vi "SVFA Zoom Power Spectrum (N Ch).vi"(0 "scaled signals [EU]":waveform(dbl)[](array[waveform]), 3 "zoom settings":T2={"frequency range"={"start frequency"=1000.0, "stop frequency"=2000.0}, "window"=1, "number of lines"=400, "% overlap"=0.0} {"% overlap" min=0.0 format="%.2f"; "number of lines" min=2; "window" items=["None ", "Hanning", "Hamming", "Blackman-Harris", "Exact Blackman", "Blackman", "Flat Top", "4 Term B-Harris ", "7 Term B-Harris", "Low Sidelobe"]; "frequency range"."stop frequency" min=0.0 format="%.2f"; "frequency range"."start frequency" min=0.0 format="%.2f"}, 4 "dB On (T)":bool=TRUE, 5 "error in (no error)":errorcluster, 7 "averaging parameters":T1={"averaging mode"=enum."No averaging", "weighting mode"=enum."Exponential", "number of averages"=10, "linear mode"=enum."One shot"} {"number of averages" min=1 step=1}, 9 "restart averaging (F)":bool) -> (11 "averaging done":bool, 12 "new spectrum available":bool, 13 "averages completed":dbl, 14 "power spectra [dB EU]":cluster{"f0":dbl, "df":dbl, "magnitude":dbl[]}[](array[cluster]) {"magnitude" format="%.2p"; "df" format="%.2p"; "f0" format="%.2p"}, 15 "unit labels":string[](array[string]), 18 "spectrum info":T3[](array[typedef]) {"x-axis units" items=["Time (s)"=0, "Frequency-CB (Hz)"=1, "Frequency-CPB (Hz)"=1248, "Frequency-Arbitrary (Hz)"=2357, "Quefrency (s)"=2, "Revolutions (rev)"=3, "Order"=4, "Speed (RPM)"=11, "Speed (rad/s)"=21, "Index"=65535]; "weighting filter" items=["Linear", "A-weighting", "B-weighting", "C-weighting", "ITU-R 468-4", "Dolby", "CCITT", "C-message", "Wb", "Wc", "Wd", "We", "Wf", "Wh", "Wj", "Wk", "Wm", "AES17 20 kHz lowpass", "AES17 40 kHz lowpass", "AES17 20 kHz highpass", "AES17 40 kHz highpass"]; "dB reference [EU]" format="%.2f"; "engineering units" items=["custom..."=0, "V"=1, "A"=21, "C"=30, "pC"=31, "s"=32, "-"=29, "Pa"=2, "N"=20, "g"=3, "m/s^2"=4, "m/s"=5, "m"=6, "mm/s"=12, "mm"=13, "micron/s"=14, "micron"=15, "in/s^2"=7, "in/s"=8, "in"=9, "mil/s"=10, "mil"=11, "rad/s^2"=16, "rad/s"=17, "rad"=18, "deg/s^2"=26, "deg/s"=27, "deg"=28, "RPM"=22, "cycle/s^2"=23, "Hz"=24, "cycle"=25, "strain"=19]; "spectral info"."window" items=["None "=0, "Hanning"=1, "Hamming"=2, "Blackman-Harris"=3, "Exact Blackman"=4, "Blackman"=5, "Flat Top"=6, "4 Term B-Harris "=7, "7 Term B-Harris"=8, "Low Sidelobe"=9, "Force - Exponential"=10, "Gaussian"=62]}, 19 "error out":errorcluster)   [LabVIEW 2017]
doc: "Computes the zoom power spectrum of <B>scaled signal [EU]</B> and <B>zoom settings</B>. Data accumulates each time this VI is called. However, it returns a new spectrum only when sufficient data accumulates. Indicators and subsequent processing should only be called when <B>new spectrum available</B> is TRUE. Wire data to the <B>scaled signal [EU]</B> input to determine the polymorphic instance to use or manually select the instance."
uses:
  <vilib>/addons/_NISVFA/_Shared subVIs/Controls/svc_Spectrum Info.ctl
  <vilib>/addons/_NISVFA/_Shared subVIs/Controls/svc_X-Axis Units.ctl
  <vilib>/addons/_NISVFA/_Shared subVIs/Controls/svc_Spectrum Type.ctl
  <vilib>/addons/_NISVFA/_Shared subVIs/Controls/svc_Engineering Units Text Ring.ctl
  <vilib>/addons/_NISVFA/_Shared subVIs/Controls/svc_Weighting Filter Text Ring.ctl
  <vilib>/addons/_NISVFA/_Shared subVIs/Controls/svc_Complimentary Spectrum Units.ctl
  <vilib>/addons/_NISVFA/_Shared subVIs/Spectrum Info/svfa_Build Spectrum Info.vi
  <vilib>/addons/_NISVFA/_Shared subVIs/Spectrum Averaging/svfa_Reset Averaging State Info.vi
  <vilib>/addons/_NISVFA/_Shared subVIs/Spectrum Averaging/svfa_Average Array with Avg Checks (complex) No State.vi
  <vilib>/addons/_NISVFA/_Shared subVIs/Common/svc_Complex to Mag2 Array.vi
  <vilib>/addons/_NISVFA/_Shared subVIs/Spectrum Averaging/svfa_Average Array with Avg Checks (real) No State.vi
  <vilib>/addons/_NISVFA/_Shared subVIs/Common/svc_Get SV Channel Info.vi
  <vilib>/addons/_NISVFA/_Shared subVIs/Common/svc_Spectrum Units.vi
  <vilib>/addons/_NISVFA/_Shared subVIs/Spectrum Averaging/svfa_Average Array (complex) No State.vi
  <vilib>/addons/_NISVFA/_Shared subVIs/Spectrum Averaging/svfa_Average Array (real) No State.vi
  <vilib>/addons/_NISVFA/_Shared subVIs/Spectrum Averaging/svfa_No Average Array (complex).vi
  <vilib>/addons/_NISVFA/_Shared subVIs/Spectrum Averaging/svfa_Average Array (complex).vi
  <vilib>/addons/_NISVFA/_Shared subVIs/Spectrum Averaging/svfa_No Average Array (real).vi
  <vilib>/addons/_NISVFA/_Shared subVIs/Spectrum Averaging/svfa_Average Array (real).vi
  <vilib>/addons/_NISVFA/_Shared subVIs/Spectrum Averaging/svfa_Peak Hold Array.vi
  <vilib>/addons/_NISVFA/_Shared subVIs/Common/svc_Get Weighting Enum and Labels.vi
  <vilib>/addons/_NISVFA/_Shared subVIs/Common/svc_Unit Label Lexical Class.vi
  <vilib>/addons/_NISVFA/_Shared subVIs/Common/svc_Engineering Units to Unit Label.vi
  <vilib>/addons/_NISVFA/_Shared subVIs/Common/svc_Format Value (DBL).vi
  <vilib>/addons/_NISVFA/_Shared subVIs/Common/svc_Channel Info to Spectrum Info.vi
  <vilib>/addons/_NISVFA/_Shared subVIs/Common/svc_Unit Label to Engineering Units.vi
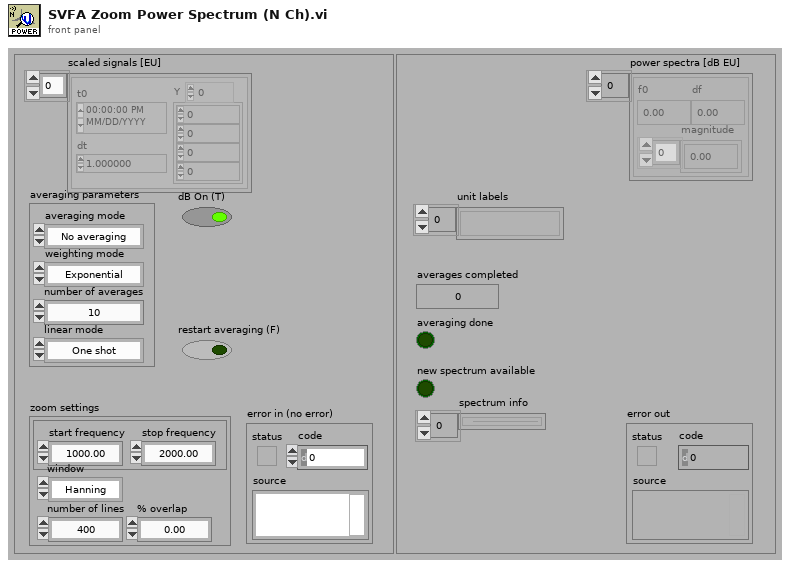
[diagram p1: front panel]
types:
  T1 = cluster{"averaging mode":enum16{"No averaging", "Vector averaging", "RMS averaging", "Peak hold"}, "weighting mode":enum16{"Linear", "Exponential"}, "number of averages":u32, "linear mode":enum16{"One shot", "Auto restart"}}
  T2 = cluster{"frequency range":cluster{"start frequency":dbl, "stop frequency":dbl}, "window":u16, "number of lines":i32, "% overlap":dbl}
  T3 = typedef "svc_Spectrum Info.ctl" = cluster{"channel name":string, "description":string, "x-axis units":T4, "spectral info":cluster{"spectrum type":T5, "linear/dB":enum16{"linear", "dB"}, "window":u16, "window size":i32, "FFT size":i32}, "engineering units":T6, "custom label":string, "dB reference [EU]":dbl, "peak units":enum16{"rms", "peak", "peak-peak"}, "weighting filter":T7, "spectral density?":bool, "unit label":string, "spectrum skewed?":bool, "complimentary spectrum units":T8}
  T4 = typedef "svc_X-Axis Units.ctl" = u16
  T5 = typedef "svc_Spectrum Type.ctl" = enum16{"FFT Spectrum [complex]", "Amplitude [Magnitude]", "Power [Magnitude^2]", "Cross Spectrum [complex]", "Frequency Response [Complex]"}
  T6 = typedef "svc_Engineering Units Text Ring.ctl" = u16
  T7 = typedef "svc_Weighting Filter Text Ring.ctl" = u16
  T8 = typedef "svc_Complimentary Spectrum Units.ctl" = enum16{"none", "radians", "degrees", "cycles", "imaginary"}
  T9 = enum16{"Restart processing", "Continue processing", "Skip processing"}
  T10 = enum16{"No averaging", "Vector averaging", "RMS averaging", "Peak hold"}
  T11 = cluster{"complex FFT":cdb[], "real FFT":dbl[], "f0":dbl, "df":dbl, "averages completed":dbl, "averaging parameters":cluster{"averaging mode":enum16{"No averaging", "Vector averaging", "RMS averaging", "Peak hold"}, "weighting mode":enum16{"Linear", "Exponential"}, "number of averages":u32, "linear mode":enum16{"One shot", "Auto restart"}}}[]
  T12 = cluster{"zoom settings":cluster{"center frequency":dbl, "zoom":i32, "trim":dbl}, "FFT settings":cluster{"window":enum16{"None ", "Hanning", "Hamming", "Blackman-Harris", "Exact Blackman", "Blackman", "Flat Top", "4 Term B-Harris ", "7 Term B-Harris", "Low Sidelobe"}, "window size":i32, "FFT size":i32, "%overlap":dbl}}
  T13 = cluster{"complex FFT":cdb[], "real FFT":dbl[], "f0":dbl, "df":dbl, "averages completed":dbl, "averaging parameters":cluster{"averaging mode":enum16{"No averaging", "Vector averaging", "RMS averaging", "Peak hold"}, "weighting mode":enum16{"Linear", "Exponential"}, "number of averages":u32, "linear mode":enum16{"One shot", "Auto restart"}}}
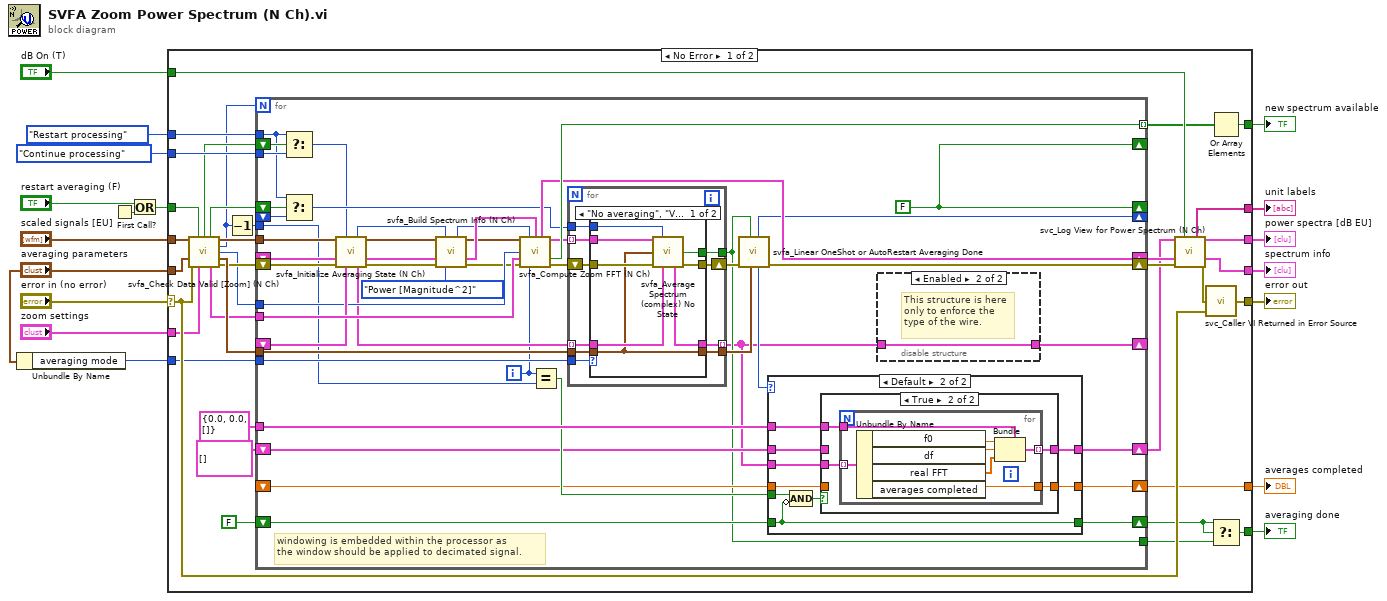
[diagram p0: block diagram]
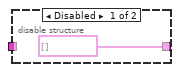
[diagram p2: hidden frame]
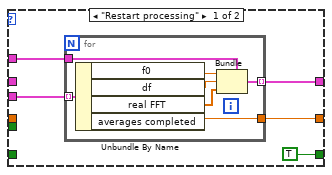
[diagram p3: hidden frame]
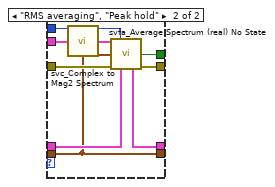
[diagram p5: hidden frame]
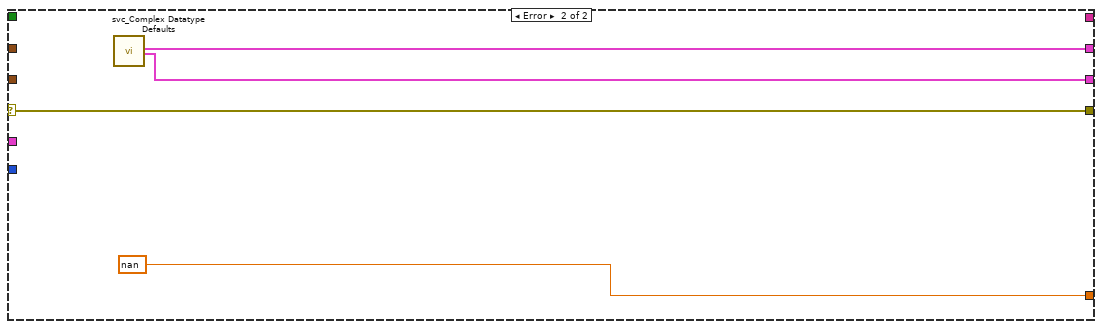
[diagram p6: hidden frame]
diagram:
  n1 = Unbundle By Name("averaging parameters") -> ("averaging mode"=w1:T10)
  n2 = First Call?() -> (First Call?: T/F=w7:bool)
  n3 = Or(x="restart averaging (F)", y=w7) -> (x .or. y?=w5:bool)
  n4 = case shown="No Error" "error in (no error)" {
    selector: "error in (no error)" -> [w37 w167]
    tunnel: w5 -> [w31 _]
    tunnel: [w23 nan ("Averaged So-far")] -> w18
    tunnel: [w34 _] -> w17
    tunnel: [w52 w164] -> w13
    tunnel: [w46 w167] -> w16
    tunnel: "averaging parameters" -> [w47 _]
    tunnel: "zoom settings" -> [w36 _]
    tunnel: "scaled signals [EU]" -> [w53 _]
    tunnel: [w50 _] -> w12
    tunnel: "dB On (T)" -> [w49 _]
    tunnel: [w48 w165] -> w11
    tunnel: [w22 _] -> w9
    tunnel: T9."Restart processing" ("processing control in") -> [w33 _]
    tunnel: T9."Continue processing" ("processing control in") -> [w32 _]
    tunnel: w1 -> [w29 _]
    frame No Error {
      n5 = call <vilib>:"svfa_Check Data Valid [Zoom] (N Ch).vi"("scaled signals [EU]"=w53, "restart averaging (F)"=w31, "averaging parameters"=w47, "error in (no error)"=w37, "zoom settings"=w36) -> ("reset processing"=w30:bool, "restart averaging"=w38:bool, "dup scaled signals"=w44:waveform(dbl)[], "iterations"=w28:i32, "maximum block size"=w35:i32, "dup averaging parameters"=w41:T1, "zoom FFT settings"=w39:T12, "error out"=w40:errorcluster)  [unwired: 3 in]
      n6 = Decrement(x=w28) -> (x-1=w27:i32)
      n7 = for {
        N: w28 -> [_]
        tunnel: [w97] -> w45 mode=indexing
        tunnel: w39 -> [w99]
        tunnel: w44 -> [w100]
        tunnel: [w56] -> w21
        shift-left: _ -> [w93]
        shift-right: [w54] -> _
        shift-right: [w95] -> w43
        shift-left: _ -> [w94]
        tunnel: w41 -> [w92]
        shift-right: [w60] -> _
        shift-left: _ -> [w91]
        shift-right: [w67] -> _
        shift-left: w38 -> [w89]
        tunnel: w35 -> [w88]
        shift-right: [w96] -> w42
        shift-left: w40 -> [w98]
        tunnel: w33 -> [w85]
        tunnel: w32 -> [w87]
        tunnel: w29 -> [w83]
        tunnel: w27 -> [w68]
        shift-right: [w67] -> _
        shift-left: w30 -> [w86]
        tunnel: cluster{"f0":dbl, "df":dbl, "real FFT":dbl[]} {"f0"=0.0, "df"=0.0, "real FFT"=[]} ("cluster") -> [w66]
        shift-right: [w64] -> w23
        shift-left: _ -> [w61]
        shift-right: [w63] -> w20
        shift-left: FALSE ("restart averaging") -> [w62]
        shift-right: [w58] -> w24
        shift-left: cluster{"f0":dbl, "df":dbl, "real FFT":dbl[]}[] [] -> [w57]
        i -> [w59]
        w67 = FALSE ("restart averaging")
        # "windowing is embedded within the processor as \nthe window should be applied to decimated signal."
        n8 = Select(t=w85, s=w86, f=w87) -> (s? t:f=w84:T9)
        n9 = Select(t=w85, s=w89, f=w91) -> (s? t:f=w90:T9)
        n10 = call <vilib>:"svfa_Initialize Averaging State (N Ch).vi"("Windowed Waveform(s)"=w100, "processing control in"=w84, "spectra info in"=w94, "error in (no error)"=w98, "state info"=w93) -> ("processing control out"=w77:T9, "Windowed Waveform(s)"=w76:waveform(dbl)[], "spectra info out"=w74:T3[], "state info"=w73:T11, "error out"=w75:errorcluster)  [unwired: 6 in]
        n11 = call <vilib>:"svfa_Build Spectrum Info (N Ch).vi"("scaled signal(s)"=w76, "processing control in"=w77, "spectra info in"=w74, "error in (no error)"=w75, "spectrum type"=svc_Spectrum_Type."Power [Magnitude^2]") -> ("dup processing control"=w70:T9, "dup scaled signals"=w79:waveform(dbl)[], "spectra info out"=w81:T3[], "error out"=w71:errorcluster)  [unwired: 7 in]
        n12 = call <vilib>:"svfa_Compute Zoom FFT (N Ch).vi"("scaled signals [EU]"=w79, "processing control"=w70, "spectra info in"=w81, "maximum block size"=w88, "zoom FFT settings"=w99, "error in (no error)"=w71, "iteration"=w59) -> ("spectra info out"=w95:T3[], "FFT spectra"=w78:cluster{"f0":dbl, "df":dbl, "spectrum":cdb[]}[], "spectrum ready"=w97:bool, "error out"=w80:errorcluster)  [unwired: 4 in, 1 out]
        n13 = Equal?(x=w59, y=w68) -> (x = y?=w65:bool)
        n14 = for {
          tunnel: [w146] -> w56
          tunnel: w78 -> [w145] mode=indexing
          tunnel: w90 -> [w142]
          tunnel: w92 -> [w141]
          tunnel: w83 -> [w140]
          tunnel: w73 -> [w139] mode=indexing
          tunnel: [w138] -> w55 mode=indexing
          shift-right: [w143] -> w82
          shift-left: w80 -> [w144]
          tunnel: [w137] -> w69
          n15 = case shown="\"No averaging\", \"Vector averaging\"" w140 {
            tunnel: w141 -> [w147 w155]
            tunnel: [w152 w161] -> w143
            tunnel: [w151 w162] -> w146
            tunnel: w145 -> [w154 w160]
            tunnel: w144 -> [w153 w163]
            tunnel: w142 -> [w150 w158]
            tunnel: w139 -> [w149 w156]
            tunnel: [w148 w157] -> w138
            tunnel: [w147 w155] -> w137
            frame "No averaging", "Vector averaging" {
              n16 = call <vilib>:"svfa_Average Spectrum (complex) No State.vi"("spectrum"=w154, "processing control"=w150, "averaging parameters"=w147, "error in (no error)"=w153, "averaging state info in"=w149) -> ("averaging done"=w151:bool, "averaging state info out"=w148:T13, "error out"=w152:errorcluster)  [unwired: 5 in, 3 out]
            }
            frame "RMS averaging", "Peak hold" {
              n17 = call <vilib>:"svc_Complex to Mag2 Spectrum.vi"("complex spectrum"=w160) -> ("power spectrum"=w159:cluster{"f0":dbl, "df":dbl, "spectrum":dbl[]})  [unwired: 4 in]
              n18 = call <vilib>:"svfa_Average Spectrum (real) No State.vi"("spectrum"=w159, "processing control"=w158, "averaging parameters"=w155, "error in (no error)"=w163, "averaging state info in"=w156) -> ("averaging done"=w162:bool, "averaging state info out"=w157:T13, "error out"=w161:errorcluster)  [unwired: 5 in, 3 out]
            }
          }
        }
        n19 = call <vilib>:"svfa_Linear OneShot or AutoRestart Averaging Done.vi"("averaging parameters"=w69, "averaging done"=w56, "error in (no error)"=w82) -> ("error out"=w96:errorcluster, "processing control"=w60:T9)  [unwired: 7 in]
        n20 = case shown="Default" w60 {
          tunnel: w55 -> [w107 w123]
          tunnel: [TRUE ("restart averaging") w118] -> w63
          tunnel: [w105 w122] -> w58
          tunnel: w62 -> [_ w118]
          tunnel: w65 -> [_ w121]
          tunnel: w66 -> [w104 w120]
          tunnel: [w103 w117] -> w64
          tunnel: w61 -> [_ w116]
          tunnel: w57 -> [_ w115]
          frame "Restart processing" {
            n21 = for {
              tunnel: w107 -> [w111] mode=indexing
              tunnel: [w110] -> w105 mode=indexing
              tunnel: w104 -> [w109]
              tunnel: [w108] -> w103
              n22 = Unbundle By Name(w111) -> ("f0"=w114:dbl, "df"=w113:dbl, "real FFT"=w112:dbl[], "averages completed"=w108:dbl)
              n23 = Bundle(cluster=w109, "f0"=w114, "df"=w113, "real FFT"=w112) -> (w110:cluster{"f0":dbl, "df":dbl, "real FFT":dbl[]})
            }
          }
          frame Default {
            n24 = Compound Arithmetic op=AND(w121, invert w118) -> (w119:bool)
            n25 = case shown="True" w119 {
              tunnel: w123 -> [_ w129]
              tunnel: [w124 w128] -> w122
              tunnel: w120 -> [_ w127]
              tunnel: [w125 w126] -> w117
              tunnel: w116 -> [w125 _]
              tunnel: w115 -> [w124 _]
              frame False {
              }
              frame True {
                n26 = for {
                  tunnel: w129 -> [w133] mode=indexing
                  tunnel: [w132] -> w128 mode=indexing
                  tunnel: w127 -> [w131]
                  tunnel: [w130] -> w126
                  n27 = Unbundle By Name(w133) -> ("f0"=w136:dbl, "df"=w135:dbl, "real FFT"=w134:dbl[], "averages completed"=w130:dbl)
                  n28 = Bundle(cluster=w131, "f0"=w136, "df"=w135, "real FFT"=w134) -> (w132:cluster{"f0":dbl, "df":dbl, "real FFT":dbl[]})
                }
              }
            }
          }
        }
        n29 = disable-structure shown="Enabled" {
          disable-tunnel: [T11 [] w102] -> w54
          disable-tunnel: w55 -> [_ w102]
          frame Disabled {
          }
          frame Enabled {
            # "This structure is here\nonly to enforce the\ntype of the wire."
          }
        }
      }
      n30 = call <vilib>:"svc_Log View for Power Spectrum (N Ch).vi"("Power Spectra [EU^2 rms]"=w24, "dB On (F)"=w49, "spectra info in"=w43, "error in (no error)"=w42) -> ("unit label(s)"=w50:string[], "Power Spectra [EU^2 rms]"=w52:cluster{"f0":dbl, "df":dbl, "spectrum":dbl[]}[], "spectra info out"=w48:T3[], "error out"=w51:errorcluster)  [unwired: 8 in]
      n31 = call <vilib>:"svc_Caller VI Returned in Error Source.vi"("warning input to caller"=w37, "error in (no error)"=w51) -> ("error out"=w46:errorcluster)  [unwired: 3 in]
      n32 = Or Array Elements(Boolean array=w45) -> (logical OR=w34:bool)
      n33 = Select(t=w20, s=w20, f=w21) -> (s? t:f=w22:bool)
    }
    frame Error {
      n34 = call <vilib>:"svc_Complex Datatype Defaults.vi"() -> ("empty array of spectra"=w164:cluster{"f0":dbl, "df":dbl, "magnitude":dbl[]}[], "empty array of spectrum info"=w165:T3[])  [unwired: 11 in, 7 out]
    }
  }
  "averages completed" <- w18
  "new spectrum available" <- w17
  "error out" <- w16
  "power spectra [dB EU]" <- w13
  "unit labels" <- w12
  "spectrum info" <- w11
  "averaging done" <- w9
